vi "Test Autostop Nested Actors.vi"(11 "Test Case In":refnum<class "AF Test.lvclass">) -> (0 "error out":errorcluster, 3 "Test Case Out":refnum<class "AF Test.lvclass">)   [LabVIEW 2020, in "AF Test.lvclass"]
uses:
  AF Test.lvclass
  C:/Program Files (x86)/National Instruments/LabVIEW 2020/vi.lib/Astemes/LUnit/Test Case.lvclass
  <vilib>/Astemes/LUnit/Test Case.lvclass/Test Case.ctl
  4993e8ee-a06a-463a-9684-69129f64d5ce.vi
  <vilib>/Astemes/LUnit/Core/LUnit Test Case/Private/Append Pass Result.vi
  <vilib>/Astemes/LUnit/Core/LUnit Test Case/Private/Append Fail Result.vi
  4993e8ee-a06a-463a-9684-69129f64d5ce.vi/9c5d11cd-9439-4240-a1ee-d9baace9c924.vi
  <vilib>/Astemes/LUnit/Core/LUnit Test Case/Private/Run In UI.vi
  <vilib>/Utility/error.llb/Clear Errors.vi
  AF Test.lvclass/AF Test.ctl
  Test Harness/Actor with Nesteds/Actor with Nesteds/Actor with Nesteds.lvclass
  ActorFramework/Actor/Actor.lvclass
  ActorFramework/Message Queue/Message Queue.lvclass
  Test Harness/Actor with Nesteds/Actor with Nesteds Messages/Stop Nested Actors Msg/Stop Nested Actors Msg.lvclass
  ActorFramework/Stop Msg/Stop Msg.lvclass
  ActorFramework/Message Dequeuer/Message Dequeuer.lvclass
  C:/Users/Neil/Documents/actor-framework/Core/ActorFramework/Actor/Actor.lvclass
  C:/Users/Neil/Documents/actor-framework/Core/Testing/Test Harness/Actor with Nesteds/Actor with Nesteds/Actor with Nesteds.lvclass
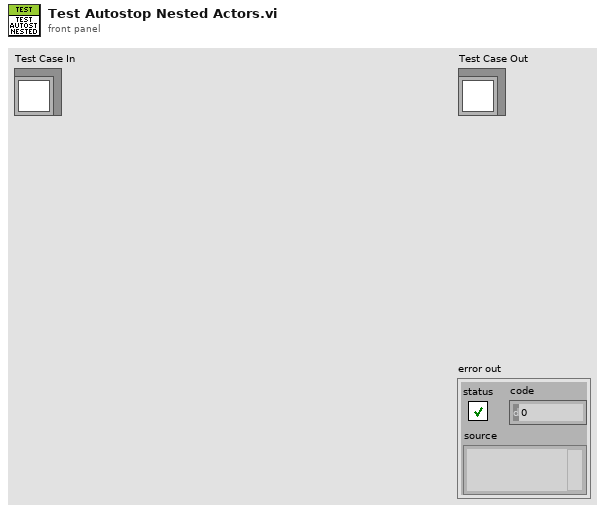
[diagram p1: front panel]
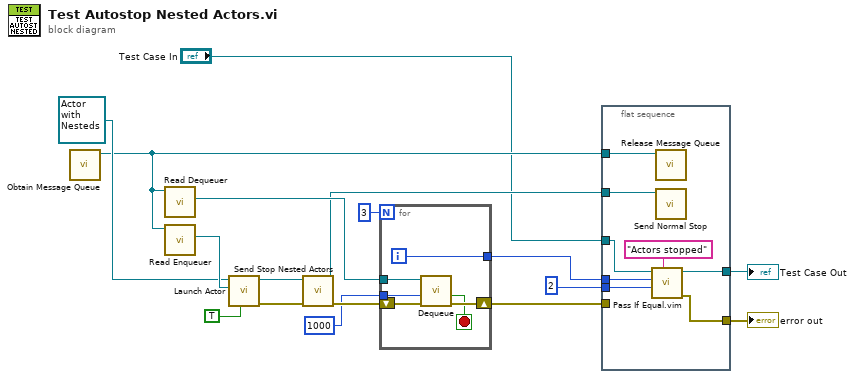
[diagram p0: block diagram]
diagram:
  n1 = call "Obtain Message Queue.vi"() -> ("Message Queue"=w9:refnum<class "Message Queue.lvclass">)  [unwired: 10 in, 1 out]
  n2 = call "Read Dequeuer.vi"("Message Queue"=w9) -> ("Message Dequeuer"=w12:refnum<class "Message Dequeuer.lvclass">)  [unwired: 10 in]
  n3 = call "Read Enqueuer.vi"("Message Queue"=w9) -> ("Message Enqueuer"=w17:refnum<class "Message Enqueuer.lvclass">)  [unwired: 10 in]
  n4 = call "Launch Actor.vi"("Open Actor Core front panel? (F)"=TRUE, "Actor-to-Caller Enqueuer"=w17, "Actor"=refnum<class "Actor with Nesteds.lvclass"> refnum ("Actor with Nesteds.lvlib:Actor with Nesteds.lvclass")) -> ("error out"=w16:errorcluster, "Caller-To-Actor Enqueuer"=w15:refnum<class "Message Enqueuer.lvclass">)  [unwired: 7 in]
  n5 = call "Send Stop Nested Actors.vi"("error in (no error)"=w16, "Message Enqueuer"=w15) -> ("error out"=w14:errorcluster, "Message Enqueuer out"=w4:refnum<class "Message Enqueuer.lvclass">)  [unwired: 8 in]
  n6 = for {
    N: 3 -> [_]
    tunnel: u32 1000 ("milliseconds to wait") -> [w22]
    tunnel: w12 -> [w21]
    shift-right: [w20] -> w11
    shift-left: w14 -> [w23]
    tunnel: [w18] -> w6
    i -> [w18]
    stop <- w19 stop-if-true
    n7 = call "Dequeue.vi"("error in (no error)"=w23, "timeout in ms (-1)"=w22, "Message Dequeuer in"=w21) -> ("error out"=w20:errorcluster, "timed out?"=w19:bool)  [unwired: 4 in, 3 out]
  }
  n8 = flat-sequence {
    tunnel: w11 -> [_]
    tunnel: w9 -> [w31]
    tunnel: w6 -> [w25]
    tunnel: 2 -> [w24]
    tunnel: w4 -> [w30]
    tunnel: "Test Case In" -> [w29]
    tunnel: [w28] -> w2
    tunnel: [w27] -> w1
    frame #0 {
      n9 = call "Pass If Equal.vim"("Description"="Actors stopped" ("Label (VI Title)"), "Actual"=w24, "Expected"=w25, "LUnit Test Case In"=w29) -> ("error out"=w28:errorcluster, "LUnit Test Case Out"=w27:refnum<class "AF Test.lvclass">)  [unwired: 6 in]
      n10 = call "Release Message Queue.vi"("Message Queue"=w31) -> ()  [unwired: 9 in, 2 out]
      n11 = call "Send Normal Stop.vi"("Message Enqueuer"=w30) -> ()  [unwired: 10 in, 1 out]
    }
  }
  "error out" <- w2
  "Test Case Out" <- w1
